vi "HIOKI PW3390 Conf Beep.vi"(4 "Error Out (F: Off)":bool, 6 "OPC query (T: ON)":bool=TRUE, 7 "Set/Query (F: Set)":bool, 8 "error in (no error)":errorcluster, 10 "Beep (T: ON)":bool=TRUE, 11 "VISA Resource":refnum<visa-resource-name>) -> (0 "error out":errorcluster, 2 "Beep out":bool=TRUE, 3 "VISA Resource out":refnum<visa-resource-name>)   [LabVIEW 2009]
doc: "Set/Query\n Set: Send the setting commands for the device.\n Query: Query the setting of the device.\n\nBeep\n Sets the beep setting."
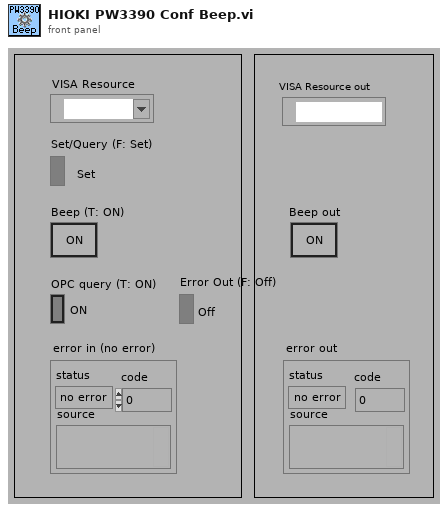
[diagram p1: front panel]
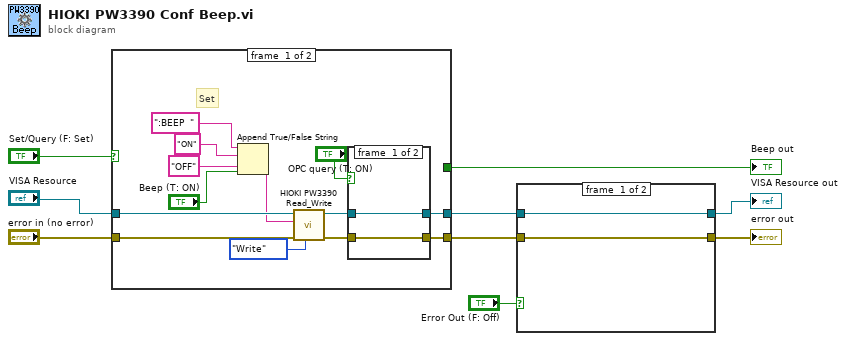
[diagram p0: block diagram]
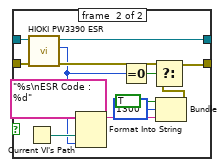
[diagram p2: hidden frame]
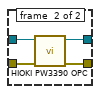
[diagram p3: hidden frame]
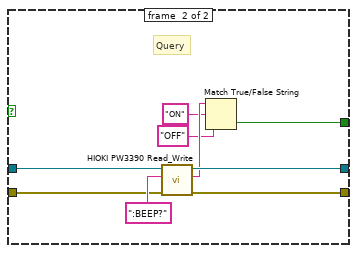
[diagram p4: hidden frame]
diagram:
  n1 = case shown="FALSE" "Set/Query (F: Set)" {
    tunnel: "error in (no error)" -> [w21 w36]
    tunnel: [w14 w34] -> w6
    tunnel: "VISA Resource" -> [w22 w35]
    tunnel: [w15 w33] -> w5
    tunnel: [_ w29] -> w1
    frame #0 {
      # "Set"
      n2 = Append True/False String(1:"Beep (T: ON)", 2:"OFF" ("false文字列"), 3:"ON" ("true文字列"), 4:":BEEP  ") -> (0:w19:string)
      n3 = call <instrlib>:"HIOKI PW3390 Read_Write.vi"("Read/Write"=enum16{"Read", "Write"}."Write", "error in (no error)"=w21, "data in"=w19, "VISA Resource"=w22) -> ("error out"=w16:errorcluster, "VISA Resource out"=w17:refnum<visa-resource-name>)  [unwired: 5 in, 1 out]
      n4 = case shown="TRUE" "OPC query (T: ON)" {
        tunnel: [w24 w28] -> w15
        tunnel: [w23 w27] -> w14
        tunnel: w17 -> [w24 w26]
        tunnel: w16 -> [w23 w25]
        frame #0 {
        }
        frame #1 {
          n5 = call <instrlib>:"HIOKI PW3390 OPC.vi"("error in (no error)"=w25, "VISA Resource"=w26) -> ("error out"=w27:errorcluster, "VISA Resource out"=w28:refnum<visa-resource-name>)  [unwired: 7 in, 1 out]
        }
      }
    }
    frame #1 {
      # "Query"
      n6 = call <instrlib>:"HIOKI PW3390 Read_Write.vi"("error in (no error)"=w36, "data in"=":BEEP?", "VISA Resource"=w35) -> ("error out"=w34:errorcluster, "data out"=w32:string, "VISA Resource out"=w33:refnum<visa-resource-name>)  [unwired: 6 in]
      n7 = Match True/False String(2:"OFF" ("false文字列"), 3:"ON" ("true文字列"), 4:w32) -> (0:w29:bool)  [unwired: 1 out]
    }
  }
  "Beep out" <- w1
  n8 = case shown="TRUE" "Error Out (F: Off)" {
    tunnel: w5 -> [w39 w52]
    tunnel: w6 -> [w38 w51]
    tunnel: [w38 w41] -> w4
    tunnel: [w39 w50] -> w2
    frame #0 {
    }
    frame #1 {
      n9 = Current VI's Path() -> (path=w48:path)
      n10 = call <instrlib>:"HIOKI PW3390 ESR.vi"("error in (no error)"=w51, "VISA Resource"=w52) -> ("error out"=w42:errorcluster, "Output Value"=w40:u8, "VISA Resource out"=w50:refnum<visa-resource-name>)  [unwired: 6 in, 1 out]
      n11 = Format Into String(format string="%s\nESR Code : %d", w48, w40) -> (resulting string=w44:string)  [unwired: 2 in, 1 out]
      n12 = Equal To 0?(x=w40) -> (x = 0?=w49:bool)
      n13 = Bundle("status"=TRUE, "code"=1300, w44) -> (w43:cluster{"status":bool, "code":i32, string})  [unwired: 1 in]
      n14 = Select(t=w42, s=w49, f=w43) -> (s? t:f=w41:errorcluster)
    }
  }
  "error out" <- w4
  "VISA Resource out" <- w2
